vi "Get_radius_from_mass.vi"(7 "Density (g/cc)":dbl, 9 "Charge":sgl, 10 "Velocity":sgl, 11 "High Voltage (MV)":sgl) -> (2 "Mass":ext, 3 "Radius":dbl)   [LabVIEW 2013]
panel:
  # "Density of Fe: \n7.874 g·cm-3"
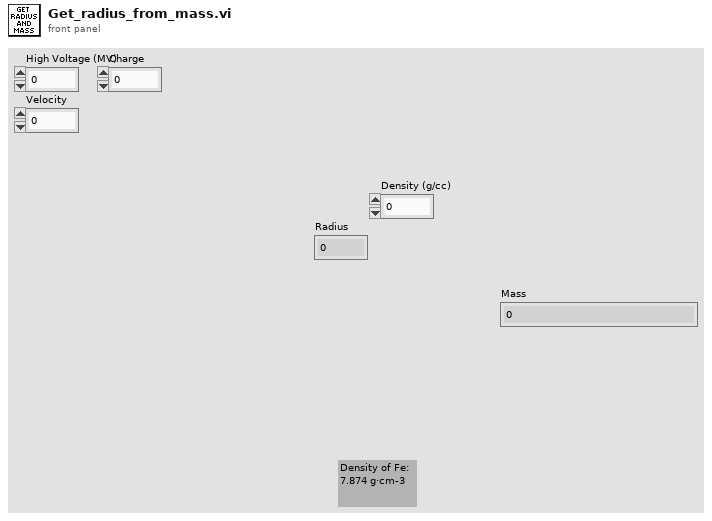
[diagram p1: front panel]
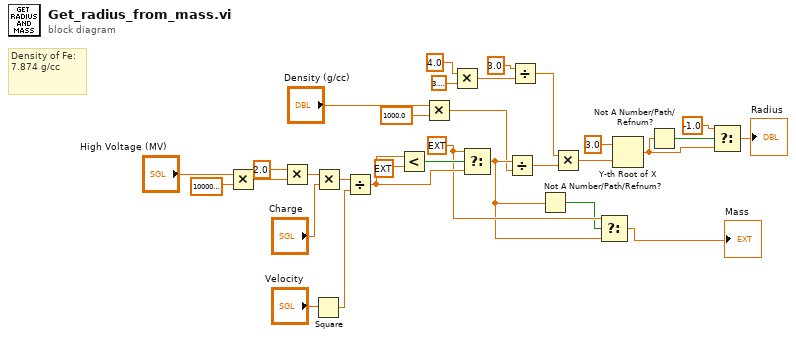
[diagram p0: block diagram]
diagram:
  w7 = ext -1.0 ("y")
  # "Density of Fe: \n7.874 g/cc"
  n1 = Multiply(x="High Voltage (MV)", y=sgl 1000000.0) -> (x*y=w10:sgl)
  n2 = Multiply(x=sgl 2.0, y=w10) -> (x*y=w18:sgl)
  n3 = Square(x="Velocity") -> (x^2=w16:sgl)
  n4 = Multiply(x=w18, y="Charge") -> (x*y=w17:sgl)
  n5 = Divide(x=w17, y=w16) -> (x/y=w13:sgl)
  n6 = Less?(x=w13, y=ext 0.0) -> (x < y?=w14:bool)
  n7 = Multiply(x="Density (g/cc)", y=1000.0) -> (x*y=w3:dbl)
  n8 = Multiply(x=4.0, y=3.141592653589793) -> (x*y=w28:dbl)
  n9 = Select(t=w7, s=w14, f=w13) -> (s? t:f=w5:ext)
  n10 = Divide(x=w5, y=w3) -> (x/y=w30:ext)
  n11 = Divide(x=3.0, y=w28) -> (x/y=w29:dbl)
  n12 = Not A Number/Path/Refnum?(number/path/refnum=w5) -> (NaN/Path/Refnum?=w6:bool)
  n13 = Multiply(x=w29, y=w30) -> (x*y=w24:ext)
  n14 = Select(t=w7, s=w6, f=w5) -> (s? t:f=→"Mass":ext)
  n15 = Y-th Root of X(1:w24, 2:3.0 ("y")) -> (0:w21:ext)
  n16 = Not A Number/Path/Refnum?(number/path/refnum=w21) -> (NaN/Path/Refnum?=w22:bool)
  n17 = Select(t=-1.0, s=w22, f=w21) -> (s? t:f=→"Radius":ext)
